vi "Add Panel.vi"(0 "Top Rack Serial Number":string, 1 "Work Order":string, 2 "Waveform":string, 3 "Frequency (MHz)":string, 4 "Bottom Rack Serial Number":string, 5 "Shelf Number":string, 6 "User":string, 7 "PartNumber":string, 8 "SubNumber":string, 9 "Voltage":string, 10 "connection information":path, 11 "System Num":u32=1 min=1 max=6) -> ()   [LabVIEW 2024]
uses:
  <vilib>/addons/database/Connection.llb/DB Tools Open Connec (Path).vi
  <vilib>/addons/database/Connection.llb/Conn Execute.vi
  <vilib>/addons/database/Recordset.llb/Rec Destroy - Connection.vi
  <vilib>/addons/database/_DB Variant To Data/Database Variant To Data.xnode
  <vilib>/addons/database/NI_Database_API.lvlib
panel:
  out "TimeStart":string
  out "Last DC_SN":string
  out "System #":u32=1 min=1 max=6
  in  "Active Positions 1":string
  in  "Active Positions 2":string
  out "Rack 2":string
  out "Rack 1":string
  in  "Deselect All 2":bool
  in  "Select All 2":bool
  in  "13":bool
  in  "14":bool
  in  "15":bool
  in  "16":bool
  in  "21":bool
  in  "22":bool
  in  "23":bool
  in  "24":bool
  in  "29":bool
  in  "30":bool
  in  "31":bool
  in  "32":bool
  in  "10":bool
  in  "11":bool
  in  "12":bool
  in  "18":bool
  in  "19":bool
  in  "20":bool
  in  "26":bool
  in  "27":bool
  in  "28":bool
  in  "1":bool
  in  "2":bool
  in  "3":bool
  in  "4":bool
  in  "5":bool
  in  "6":bool
  in  "7":bool
  in  "8":bool
  in  "9":bool
  in  "17":bool
  in  "25":bool
  in  "Deselect All 1":bool
  in  "Confirm":bool
  in  "13":bool
  in  "14":bool
  in  "15":bool
  in  "16":bool
  in  "21":bool
  in  "22":bool
  in  "23":bool
  in  "24":bool
  in  "29":bool
  in  "30":bool
  in  "31":bool
  in  "32":bool
  in  "10":bool
  in  "11":bool
  in  "12":bool
  in  "18":bool
  in  "19":bool
  in  "20":bool
  in  "26":bool
  in  "27":bool
  in  "28":bool
  in  "1":bool
  in  "2":bool
  in  "3":bool
  in  "4":bool
  in  "5":bool
  in  "6":bool
  in  "7":bool
  in  "8":bool
  in  "9":bool
  in  "17":bool
  in  "25":bool
  in  "Select All 1":bool
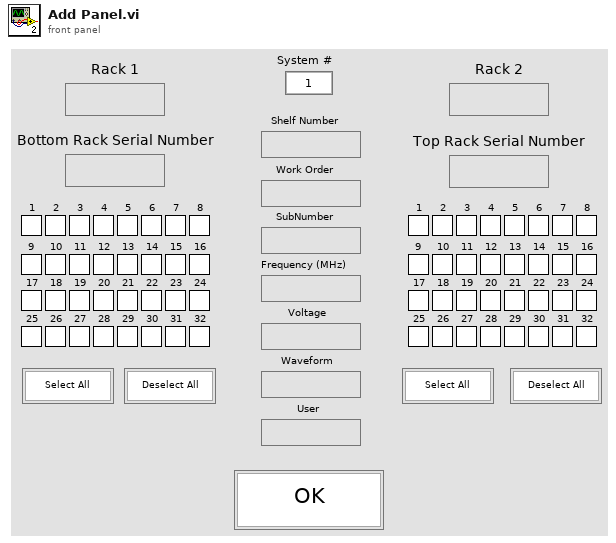
[diagram p1: front panel]
types:
  T1 = typedef "NI_Database_API.lvlib/Conn ObjectReference.ctl" = refnum<k1>
  T2 = typedef "NI_Database_API.lvlib/Rec ObjectReference.ctl" = refnum<k1>
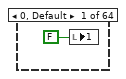
[diagram p2: hidden frame]
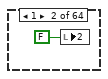
[diagram p3: hidden frame]
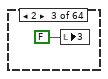
[diagram p4: hidden frame]
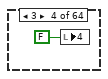
[diagram p5: hidden frame]
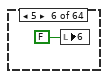
[diagram p6: hidden frame]
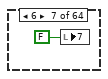
[diagram p7: hidden frame]
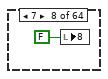
[diagram p8: hidden frame]
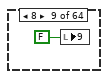
[diagram p9: hidden frame]
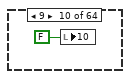
[diagram p10: hidden frame]
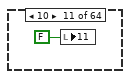
[diagram p11: hidden frame]
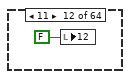
[diagram p12: hidden frame]
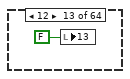
[diagram p13: hidden frame]
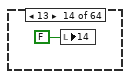
[diagram p14: hidden frame]
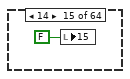
[diagram p15: hidden frame]
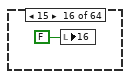
[diagram p16: hidden frame]
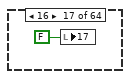
[diagram p17: hidden frame]
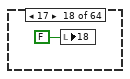
[diagram p18: hidden frame]
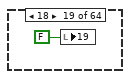
[diagram p19: hidden frame]
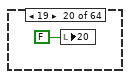
[diagram p20: hidden frame]
diagram:
  # "Any Questions? \nAsk Ben Wolford"
  n1 = flat-sequence {
    frame #0 {
      # "Opens SQL Active Systems/Racks/Positions and selects the data to show the user which positions are currently in use"
      n2 = property class="VI"() -> ("Front Panel"=w10:refnum<vi>)  [unwired: 2 in, 2 out]
      n3 = call "Display Message to User"() -> ()  [unwired: 10 in, 2 out]
      n4 = local write "Select All 1"(FALSE ("Select All")) -> ()
      n5 = local write "Confirm"(FALSE ("Confirm")) -> ()
      n6 = for {
        N: 64 -> [_]
        i -> [w13]
        n7 = case shown="4" w13 {
          frame 0, Default {
            n8 = local write "1"(FALSE ("1")) -> ()
          }
          frame 1 {
            n9 = local write "2"(FALSE ("1")) -> ()
          }
          frame 2 {
            n10 = local write "3"(FALSE ("1")) -> ()
          }
          frame 3 {
            n11 = local write "4"(FALSE ("1")) -> ()
          }
          frame 4 {
            n12 = local write "5"(FALSE ("1")) -> ()
          }
          frame 5 {
            n13 = local write "6"(FALSE ("1")) -> ()
          }
          frame 6 {
            n14 = local write "7"(FALSE ("1")) -> ()
          }
          frame 7 {
            n15 = local write "8"(FALSE ("1")) -> ()
          }
          frame 8 {
            n16 = local write "9"(FALSE ("1")) -> ()
          }
          frame 9 {
            n17 = local write "10"(FALSE ("1")) -> ()
          }
          frame 10 {
            n18 = local write "11"(FALSE ("1")) -> ()
          }
          frame 11 {
            n19 = local write "12"(FALSE ("1")) -> ()
          }
          frame 12 {
            n20 = local write "13"(FALSE ("1")) -> ()
          }
          frame 13 {
            n21 = local write "14"(FALSE ("1")) -> ()
          }
          frame 14 {
            n22 = local write "15"(FALSE ("1")) -> ()
          }
          frame 15 {
            n23 = local write "16"(FALSE ("1")) -> ()
          }
          frame 16 {
            n24 = local write "17"(FALSE ("1")) -> ()
          }
          frame 17 {
            n25 = local write "18"(FALSE ("1")) -> ()
          }
          frame 18 {
            n26 = local write "19"(FALSE ("1")) -> ()
          }
          frame 19 {
            n27 = local write "20"(FALSE ("1")) -> ()
          }
          frame 20 {
            n28 = local write "21"(FALSE ("1")) -> ()
          }
          frame 21 {
            n29 = local write "22"(FALSE ("1")) -> ()
          }
          frame 22 {
            n30 = local write "23"(FALSE ("1")) -> ()
          }
          frame 23 {
            n31 = local write "24"(FALSE ("1")) -> ()
          }
          frame 24 {
            n32 = local write "25"(FALSE ("1")) -> ()
          }
          frame 25 {
            n33 = local write "26"(FALSE ("1")) -> ()
          }
          frame 26 {
            n34 = local write "27"(FALSE ("1")) -> ()
          }
          frame 27 {
            n35 = local write "28"(FALSE ("1")) -> ()
          }
          frame 28 {
            n36 = local write "29"(FALSE ("1")) -> ()
          }
          frame 29 {
            n37 = local write "30"(FALSE ("1")) -> ()
          }
          frame 30 {
            n38 = local write "31"(FALSE ("1")) -> ()
          }
          frame 31 {
            n39 = local write "32"(FALSE ("1")) -> ()
          }
          frame 32 {
            n40 = local write "1"(FALSE ("1")) -> ()
          }
          frame 33 {
            n41 = local write "2"(FALSE ("1")) -> ()
          }
          frame 34 {
            n42 = local write "3"(FALSE ("1")) -> ()
          }
          frame 35 {
            n43 = local write "4"(FALSE ("1")) -> ()
          }
          frame 36 {
            n44 = local write "5"(FALSE ("1")) -> ()
          }
          frame 37 {
            n45 = local write "6"(FALSE ("1")) -> ()
          }
          frame 38 {
            n46 = local write "7"(FALSE ("1")) -> ()
          }
          frame 39 {
            n47 = local write "8"(FALSE ("1")) -> ()
          }
          frame 40 {
            n48 = local write "9"(FALSE ("1")) -> ()
          }
          frame 41 {
            n49 = local write "10"(FALSE ("1")) -> ()
          }
          frame 42 {
            n50 = local write "11"(FALSE ("1")) -> ()
          }
          frame 43 {
            n51 = local write "12"(FALSE ("1")) -> ()
          }
          frame 44 {
            n52 = local write "13"(FALSE ("1")) -> ()
          }
          frame 45 {
            n53 = local write "14"(FALSE ("1")) -> ()
          }
          frame 46 {
            n54 = local write "15"(FALSE ("1")) -> ()
          }
          frame 47 {
            n55 = local write "16"(FALSE ("1")) -> ()
          }
          frame 48 {
            n56 = local write "17"(FALSE ("1")) -> ()
          }
          frame 49 {
            n57 = local write "18"(FALSE ("1")) -> ()
          }
          frame 50 {
            n58 = local write "19"(FALSE ("1")) -> ()
          }
          frame 51 {
            n59 = local write "20"(FALSE ("1")) -> ()
          }
          frame 52 {
            n60 = local write "21"(FALSE ("1")) -> ()
          }
          frame 53 {
            n61 = local write "22"(FALSE ("1")) -> ()
          }
          frame 54 {
            n62 = local write "23"(FALSE ("1")) -> ()
          }
          frame 55 {
            n63 = local write "24"(FALSE ("1")) -> ()
          }
          frame 56 {
            n64 = local write "25"(FALSE ("1")) -> ()
          }
          frame 57 {
            n65 = local write "26"(FALSE ("1")) -> ()
          }
          frame 58 {
            n66 = local write "27"(FALSE ("1")) -> ()
          }
          frame 59 {
            n67 = local write "28"(FALSE ("1")) -> ()
          }
          frame 60 {
            n68 = local write "29"(FALSE ("1")) -> ()
          }
          frame 61 {
            n69 = local write "30"(FALSE ("1")) -> ()
          }
          frame 62 {
            n70 = local write "31"(FALSE ("1")) -> ()
          }
          frame 63 {
            n71 = local write "32"(FALSE ("1")) -> ()
          }
        }
      }
      n72 = property class="Pnl"(reference=w10, "Color"=u32 14869218) -> ()  [unwired: 1 in, 2 out]
      n73 = case shown="\"2\"" "Shelf Number" {
        tunnel: ["1" ("ConnectionString In") "3" ("ConnectionString In") "5" ("ConnectionString In") "7" ("ConnectionString In") "9" ("ConnectionString In") "11" ("ConnectionString In") "13" ("ConnectionString In") "15" ("ConnectionString In")] -> w7
        tunnel: ["2" ("ConnectionString In") "4" ("ConnectionString In") "6" ("ConnectionString In") "8" ("ConnectionString In") "10" ("ConnectionString In") "12" ("ConnectionString In") "14" ("ConnectionString In") "16" ("ConnectionString In")] -> w6
        frame "1", Default {
        }
        frame "2" {
        }
        frame "3" {
        }
        frame "4" {
        }
        frame "5" {
        }
        frame "6" {
        }
        frame "7" {
        }
        frame "8" {
        }
      }
      "Rack 1" <- w7
      "Rack 2" <- w6
      n74 = Get Date/Time In Seconds() -> (seconds since 1Jan1904=w3:timestamp)
      n75 = Format Date/Time String(time format string (%c)="%m/%d/%Y %I:%M %p", seconds (now)=w3) -> (date/time string=→"TimeStart":string)  [unwired: 1 in]
      "System #" <- "System Num"
    }
    frame #1 {
      n76 = while {
        stop <- w94 stop-if-true
        # "When deselect all is pressed down, set every button to inactive position"
        # "When Confirm is pressed, the current active positions are sent up to the cloud to save which ones are being used"
        # "When select all is pressed down, set every button to active position"
        n77 = event shown="[0] \"Confirm\": Value Change" {
          selector: _ -> [_ _ _ _ _]
          dyn-events: _ -> [_ _ _ _ _]
          timeout: _ -> [_ _ _ _ _]
          tunnel: [w103 _ _ _ _] -> w94
          event "Confirm": Value Change {
            n78 = event-data() -> ()  [unwired: 1 in, 1 out]
            n79 = flat-sequence {
              tunnel: [w138] -> w104
              tunnel: [w105] -> w102
              tunnel: w104 -> [w172]
              tunnel: w102 -> [w173]
              tunnel: [w175] -> w101
              tunnel: [w174] -> w100
              tunnel: w101 -> [w486]
              tunnel: w100 -> [w485]
              tunnel: [w480] -> w98
              tunnel: [w484] -> w96
              tunnel: [w599] -> w99
              tunnel: w98 -> [w599]
              tunnel: [w598] -> w97
              tunnel: w96 -> [w598]
              tunnel: w99 -> [w610]
              tunnel: w97 -> [w609]
              tunnel: [TRUE] -> w103
              frame #0 {
                # "Creates a Panel that allows users to click on individual positions to add them to the active positions"
                n80 = Build Array("1", "2", "3", "4", "5", "6", "7", "8", "9", "10", "11", "12", "13", "14", "15", "16", "17", "18", "19", "20", "21", "22", "23", "24", "25", "26", "27", "28", "29", "30", "31", "32") -> (w138:bool[])
                n81 = Build Array("1", "2", "3", "4", "5", "6", "7", "8", "9", "10", "11", "12", "13", "14", "15", "16", "17", "18", "19", "20", "21", "22", "23", "24", "25", "26", "27", "28", "29", "30", "31", "32") -> (w105:bool[])
              }
              frame #1 {
                n82 = Or Array Elements(Boolean array=w172) -> (logical OR=w177:bool)
                n83 = Or Array Elements(Boolean array=w173) -> (logical OR=w176:bool)
                n84 = Insert Into Array(array=w172, new element=w173) -> (w171:bool[])  [unwired: 1 in]
                n85 = Not(x=w177) -> (.not. x?=w175:bool)
                n86 = for {
                  N: 64 -> [_]
                  tunnel: w171 -> [w180] mode=indexing
                  shift-right: [w182] -> _
                  shift-left: "" -> [w191]
                  i -> [w187]
                  n87 = Select(t="1", s=w180, f="0") -> (s? t:f=w186:string)
                  n88 = Increment(x=w187) -> (x+1=w183:i32)
                  n89 = Concatenate Strings(w191, w186, "," ("string")) -> (w185:string)
                  n90 = Greater?(x=w183, y=32) -> (0:w181:bool)
                  n91 = case shown="True" w180 {
                    tunnel: w183 -> [_ w224]
                    tunnel: w181 -> [_ w223]
                    frame False {
                    }
                    frame True {
                      n92 = flat-sequence {
                        tunnel: w224 -> [w254]
                        tunnel: [w245] -> w216
                        tunnel: [w246] -> w214
                        tunnel: [w257] -> w212
                        tunnel: [w288] -> w210
                        tunnel: [w287] -> w208
                        tunnel: [w261] -> w206
                        tunnel: w223 -> [w253]
                        tunnel: [w245] -> w204
                        tunnel: w216 -> [w385]
                        tunnel: [w385] -> w215
                        tunnel: w214 -> [w384]
                        tunnel: [w384] -> w213
                        tunnel: w212 -> [w383]
                        tunnel: [w383] -> w211
                        tunnel: w210 -> [w382]
                        tunnel: [w382] -> w209
                        tunnel: w208 -> [w381]
                        tunnel: [w381] -> w207
                        tunnel: w206 -> [w380]
                        tunnel: [w380] -> w205
                        tunnel: w204 -> [w379]
                        tunnel: [w379] -> w203
                        tunnel: w215 -> [w395]
                        tunnel: [w395] -> w222
                        tunnel: w213 -> [w394]
                        tunnel: [w394] -> w221
                        tunnel: w211 -> [w393]
                        tunnel: [w393] -> w220
                        tunnel: w209 -> [w392]
                        tunnel: [w392] -> w219
                        tunnel: w207 -> [w391]
                        tunnel: [w391] -> w218
                        tunnel: w205 -> [w389]
                        tunnel: [w389] -> w217
                        tunnel: w203 -> [w386]
                        tunnel: w222 -> [_]
                        tunnel: w221 -> [_]
                        tunnel: w220 -> [_]
                        tunnel: w219 -> [w404]
                        tunnel: w218 -> [w405]
                        tunnel: w217 -> [w426]
                        frame #0 {
                          w243 = "," ("string")
                          # "If true, the DC_SN is checked that it abides by the format, and adds all the data displayed in the master key for the oscillator"
                          # "Master Key:\n1. DC_SN\n2. WorkOrder\n3. SystemNumber\n4. RackNumber\n5. PositionNumber\n6. RackSerialNumber\n7. TimeStart\n8. Nominal Frequency\n9. OscVoltage\n10. Waveform"
                          n93 = while {
                            tunnel: [w316] -> w246
                            stop <- w315 stop-if-true
                            n94 = flat-sequence {
                              tunnel: [w318] -> w314
                              tunnel: [w317] -> w313
                              tunnel: [w326] -> w312
                              tunnel: [w323] -> w310
                              tunnel: [w324] -> w308
                              tunnel: w313 -> [w325]
                              tunnel: w314 -> [w326]
                              tunnel: w312 -> [w370]
                              tunnel: [w370] -> w311
                              tunnel: w310 -> [w369]
                              tunnel: [w369] -> w309
                              tunnel: w308 -> [w368]
                              tunnel: w311 -> [w375]
                              tunnel: [w375] -> w316
                              tunnel: w309 -> [w372]
                              tunnel: [w373] -> w315
                              frame #0 {
                                n95 = call "Prompt User for Input"() -> ("DC_SN"=w318:string)  [unwired: 17 in, 2 out]
                                n96 = String To Byte Array(string=w318) -> (unsigned byte array=w317:u8[])
                              }
                              frame #1 {
                                n97 = Index Array(array=w325, index=0) -> (element=w319:u8)
                                n98 = Not Equal?(x=69, y=w319) -> (x != y?=w321:bool)
                                n99 = case shown="False" w321 {
                                tunnel: w326 -> [_ w347]
                                tunnel: [w327 w345] -> w324
                                tunnel: w325 -> [w330 w343]
                                tunnel: w319 -> [_ w338]
                                frame False {
                                n100 = Array Subset(array=w330, index=1) -> (w329:u8[])  [unwired: 1 in]
                                n101 = for {
                                N: 5 -> [_]
                                tunnel: w329 -> [w337] mode=indexing
                                tunnel: [w333] -> w328 mode=indexing
                                n102 = In Range and Coerce(upper limit=u8 57, x=w337, lower limit=u8 48) -> (In Range?=w334:bool)  [unwired: 1 out]
                                n103 = Not(x=w334) -> (.not. x?=w333:bool)
                                }
                                n104 = Or Array Elements(Boolean array=w328) -> (logical OR=w327:bool)
                                }
                                frame True {
                                n105 = String Length(string=w347) -> (length=w353:i32)
                                n106 = Equal?(x=u8 66, y=w338) -> (x = y?=w341:bool)
                                n107 = Equal?(x=u8 98, y=w338) -> (x = y?=w339:bool)
                                n108 = Or(x=w341, y=w339) -> (x .or. y?=w342:bool)
                                n109 = case shown="False" w342 {
                                tunnel: w343 -> [w364 w367]
                                tunnel: [w364 w365] -> w346
                                frame False {
                                }
                                frame True {
                                n110 = Array Subset(array=w367, index=1) -> (w365:u8[])  [unwired: 1 in]
                                }
                                }
                                n111 = Not Equal?(x=10, y=w353) -> (x != y?=w354:bool)
                                n112 = Array Max & Min(array=w346) -> (max value=w359:u8, min value=w358:u8)  [unwired: 2 out]
                                n113 = Index Array(array=w346, index=4) -> (element=w355:u8)
                                n114 = Less Or Equal?(x=w359, y=u8 57) -> (x <= y?=w360:bool)
                                n115 = Greater Or Equal?(x=w358, y=u8 46) -> (x >= y?=w361:bool)
                                n116 = And(x=w360, y=w361) -> (x .and. y?=w362:bool)
                                n117 = Not Equal?(x=w355, y=u8 46) -> (x != y?=w357:bool)
                                n118 = Not(x=w362) -> (.not. x?=w363:bool)
                                n119 = Or(x=w357, y=w363) -> (x .or. y?=w356:bool)
                                n120 = Or(x=w354, y=w356) -> (x .or. y?=w345:bool)
                                }
                                }
                                n121 = Not(x=w324) -> (.not. x?=w323:bool)
                              }
                              frame #2 {
                                n122 = call "Display Message to User"("Enable"=w368) -> ()  [unwired: 9 in, 2 out]
                              }
                              frame #3 {
                                n123 = Concatenate Strings("You entered " ("string"), w375, " is this correct?" ("string")) -> (w371:string)
                                n124 = call "Display Message to User"("Enable"=w372, "Message"=w371) -> ("Yes"=w374:bool)  [unwired: 8 in, 1 out]
                                n125 = And(x=w374, y=w372) -> (x .and. y?=w373:bool)
                              }
                            }
                          }
                          n126 = Random Number (0-1)() -> (number: 0 to 1=w235:dbl)
                          n127 = case shown="False" w253 {
                            tunnel: [w302 w307] -> w247
                            tunnel: w254 -> [w301 w306]
                            tunnel: [w301 w304] -> w255
                            tunnel: [w300 w303] -> w252
                            frame False {
                              n128 = local read "Bottom Rack Serial Number"() -> (w300:string)
                              n129 = local read "Rack 1"() -> (w302:string)
                            }
                            frame True {
                              n130 = Subtract(x=w306, y=32) -> (x-y=w304:i32)
                              n131 = local read "Top Rack Serial Number"() -> (w303:string)
                              n132 = local read "Rack 2"() -> (w307:string)
                            }
                          }
                          n133 = Multiply(x=51.0, y=w235) -> (x*y=w232:dbl)
                          n134 = Greater?(x=w232, y=25.0) -> (0:w230:bool)
                          n135 = case shown="True" w230 {
                            tunnel: w232 -> [w296 w299]
                            tunnel: [w296 w297] -> w231
                            frame False {
                            }
                            frame True {
                              n136 = Add(x=w299, y=7.0) -> (x+y=w297:dbl)
                            }
                          }
                          n137 = Add(x=w231, y=65.0) -> (x+y=w229:dbl)
                          n138 = local read "System Num"() -> (w289:u32)
                          n139 = Build Array(w229) -> (w228:dbl[])
                          n140 = local read "Frequency (MHz)"() -> (w269:string)
                          n141 = local read "Work Order"() -> (w295:string)
                          n142 = local read "SubNumber"() -> (w258:string)
                          n143 = local read "PartNumber"() -> (w240:string)
                          n144 = local read "Waveform"() -> (w273:string)
                          n145 = local read "TimeStart"() -> (w225:string)
                          n146 = local read "Voltage"() -> (w271:string)
                          n147 = local read "User"() -> (w249:string)
                          n148 = To Unsigned Byte Integer(number=w228) -> (unsigned 8bit integer=w227:u8[])
                          n149 = Number To Decimal String(number=w289) -> (decimal integer string=w284:string)  [unwired: 1 in]
                          n150 = Number To Decimal String(number=w255) -> (decimal integer string=w263:string)  [unwired: 1 in]
                          n151 = Concatenate Strings("'" ("string"), w247, "'" ("string")) -> (w280:string)
                          n152 = Byte Array To String(unsigned byte array=w227) -> (string=w226:string)
                          n153 = Concatenate Strings("'" ("string"), w295, "'" ("string")) -> (w257:string)
                          n154 = Concatenate Strings("'" ("string"), w258, "'" ("string")) -> (w256:string)
                          n155 = Concatenate Strings("'" ("string"), w284, "'" ("string")) -> (w283:string)
                          n156 = Concatenate Strings("'" ("string"), w263, "'" ("string")) -> (w245:string)
                          n157 = Concatenate Strings("'" ("string"), w225, "'" ("string")) -> (w294:string)
                          n158 = Concatenate Strings("'" ("string"), w269, "'" ("string")) -> (w268:string)
                          n159 = Concatenate Strings("'" ("string"), w271, "'" ("string")) -> (w270:string)
                          n160 = Concatenate Strings("'" ("string"), w273, "'" ("string")) -> (w272:string)
                          n161 = Concatenate Strings("'" ("string"), w249, "'" ("string")) -> (w248:string)
                          n162 = Concatenate Strings("'" ("string"), w240, "'" ("string")) -> (w239:string)
                          n163 = Concatenate Strings("'" ("string"), w246, "'" ("string")) -> (w261:string)
                          n164 = Concatenate Strings("UPDATE MASTER\nSET DC_SN = CONCAT(DC_SN, '" ("string"), w226, "')\nWHERE DC_SN = " ("string"), w261) -> (w287:string)
                          n165 = Concatenate Strings("INSERT INTO MASTER\nVALUES(" ("SQL Query"), w261, w243, w257, w243, w256, w243, w283, w243, w280, w243, w245, w243, w252, w243, w294, w243, w268, w243, w270, w243, w272, w243, w248, w243, w239, ");" ("string")) -> (w288:string)
                        }
                        frame #1 {
                          n166 = Wait (ms)(milliseconds to wait=u32 500) -> ()  [unwired: 1 out]
                        }
                        frame #2 {
                          n167 = Concatenate Strings("Please place DC_SN " ("Message"), w389, " into position " ("string"), w386) -> (w387:string)
                          n168 = call "Display Message to User"("Message"=w387) -> ()  [unwired: 9 in, 2 out]
                        }
                        frame #3 {
                          n169 = local read "connection information"() -> (w413:path)
                          n170 = Concatenate Strings("WHERE DC_SN = " ("SQL Query"), w426) -> (w407:string)
                          n171 = call-poly <vilib>:"DB Tools Open Connection.vi"("connection information"=w413) -> ("error out"=w414:errorcluster, "connection reference"=w417:T1)  [unwired: 7 in]
                          n172 = call <vilib>:"DB Tools Select Data.vi"("condition"=w407, "error in (no error)"=w414, "table"="MASTER", "connection reference"=w417) -> ("error out"=w412:errorcluster, "data"=w410:variant[][], "connection reference out"=w416:T1)  [unwired: 2 in]
                          n173 = xnode "Database Variant To Data"("database variant"=w410, "error in (no error)"=w412, "type"=string[][] [] ("ConnectionString In")) -> ("data"=w406:string[][], "error out"=w411:errorcluster)
                          n174 = Array Size(array=w406) -> (size(s)=w425:i32[])
                          n175 = Index Array(array=w425, index=0) -> (element=w422:i32)
                          n176 = Index Array(array=w425, index=1) -> (element=w397:i32)
                          n177 = Greater?(x=w422, y=0) -> (0:w420:bool)
                          n178 = Greater?(x=w397, y=0) -> (0:w419:bool)
                          n179 = And(x=w420, y=w419) -> (x .and. y?=w403:bool)
                          n180 = case shown="True" w403 {
                            tunnel: w416 -> [w427 w435]
                            tunnel: [w428 w430] -> w415
                            tunnel: w411 -> [w428 w434]
                            tunnel: w405 -> [_ w433]
                            tunnel: [w427 w431] -> w402
                            frame False {
                            }
                            frame True {
                              n181 = call-poly <vilib>:"DB Tools Execute Query.vi"("error in (no error)"=w434, "SQL query"=w433, "connection reference"=w435) -> ("error out"=w429:errorcluster, "recordset reference"=w432:T2)  [unwired: 5 in]
                              n182 = call-poly <vilib>:"DB Tools Free Object.vi"("error in (no error)"=w429, "recordset reference"=w432) -> ("error out"=w430:errorcluster, "connection reference"=w431:T1)  [unwired: 8 in]
                            }
                          }
                          n183 = call-poly <vilib>:"DB Tools Execute Query.vi"("error in (no error)"=w415, "SQL query"=w404, "connection reference"=w402) -> ("error out"=w400:errorcluster, "recordset reference"=w401:T2)  [unwired: 5 in]
                          n184 = call-poly <vilib>:"DB Tools Free Object.vi"("error in (no error)"=w400, "recordset reference"=w401) -> ("error out"=w398:errorcluster, "connection reference"=w399:T1)  [unwired: 8 in]
                          n185 = call <vilib>:"DB Tools Close Connection.vi"("error in (no error)"=w398, "connection reference"=w399) -> ()  [unwired: 5 in, 1 out]
                        }
                      }
                    }
                  }
                  n186 = case shown="0, Default" w183 {
                    tunnel: w185 -> [w192 w199 w202]
                    tunnel: ["" "" w202] -> w182
                    tunnel: w181 -> [_ _ _]
                    frame 64 {
                      n187 = String Length(string=w192) -> (length=w195:i32)
                      n188 = Decrement(x=w195) -> (x-1=w196:i32)
                      n189 = String Subset(string=w192, length (rest)=w196) -> (substring=w194:string)  [unwired: 1 in]
                      n190 = local write "Active Positions 2"(w194) -> ()
                    }
                    frame 32 {
                      n191 = String Length(string=w199) -> (length=w200:i32)
                      n192 = Decrement(x=w200) -> (x-1=w201:i32)
                      n193 = String Subset(string=w199, length (rest)=w201) -> (substring=w198:string)  [unwired: 1 in]
                      n194 = local write "Active Positions 1"(w198) -> ()
                    }
                    frame 0, Default {
                    }
                  }
                }
                n195 = Not(x=w176) -> (.not. x?=w174:bool)
              }
              frame #2 {
                n196 = Or(x=w486, y=w485) -> (x .or. y?=w487:bool)
                n197 = local read "connection information"() -> (w482:path)
                n198 = call-poly <vilib>:"DB Tools Open Connection.vi"("connection information"=w482) -> ("error out"=w483:errorcluster, "connection reference"=w481:T1)  [unwired: 7 in]
                n199 = case shown="True" w487 {
                  tunnel: w486 -> [_ w497]
                  tunnel: w483 -> [w489 w495]
                  tunnel: [w489 w490] -> w484
                  tunnel: w481 -> [w488 w496]
                  tunnel: [w488 w493] -> w480
                  frame False {
                  }
                  frame True {
                    n200 = case shown="False" w497 {
                      tunnel: [w510 w560] -> w494
                      frame False {
                        n201 = local read "System Num"() -> (w498:u32)
                        n202 = local read "Rack 2"() -> (w503:string)
                        n203 = Fract/Exp String To Number(string=w503) -> (number=w502:dbl)  [unwired: 3 in, 1 out]
                        n204 = Number To Decimal String(number=w498) -> (decimal integer string=w499:string)  [unwired: 1 in]
                        n205 = case shown="4" w502 {
                          tunnel: [w516 w520 w524 w528 w532 w537 w540 w544] -> w501
                          tunnel: w499 -> [w517 w521 w525 w529 w533 w536 w541 w545]
                          frame 2, Default {
                            n206 = Concatenate Strings("A", w517, ".2") -> (w516:string)
                          }
                          frame 4 {
                            n207 = Concatenate Strings("A", w521, ".4") -> (w520:string)
                          }
                          frame 6 {
                            n208 = Concatenate Strings("A", w525, ".6") -> (w524:string)
                          }
                          frame 8 {
                            n209 = Concatenate Strings("A", w529, ".8") -> (w528:string)
                          }
                          frame 10 {
                            n210 = Concatenate Strings("A", w533, ".10") -> (w532:string)
                          }
                          frame 12 {
                            n211 = Concatenate Strings("A", w536, ".12") -> (w537:string)
                          }
                          frame 14 {
                            n212 = Concatenate Strings("A", w541, ".14") -> (w540:string)
                          }
                          frame 16 {
                            n213 = Concatenate Strings("A", w545, ".16") -> (w544:string)
                          }
                        }
                        n214 = local read "Top Rack Serial Number"() -> (w504:string)
                        n215 = Get Date/Time In Seconds() -> (seconds since 1Jan1904=w511:timestamp)
                        n216 = Format Date/Time String(time format string (%c)="%m/%d/%Y %I:%M %p", seconds (now)=w511) -> (date/time string=w512:string)  [unwired: 1 in]
                        n217 = Concatenate Strings("'" ("string"), w512, "'" ("string")) -> (w506:string)
                        n218 = Concatenate Strings("UPDATE MASTER\nSet TimeStart = " ("string"), w506, ", RackSerialNumber = " ("string"), w504, "WHERE RackNumber = " ("string"), w503, " AND DC_SN = '" ("string"), w501, "'" ("string")) -> (w510:string)
                      }
                      frame True {
                        n219 = local read "System Num"() -> (w549:u32)
                        n220 = local read "Rack 1"() -> (w553:string)
                        n221 = Fract/Exp String To Number(string=w553) -> (number=w552:dbl)  [unwired: 3 in, 1 out]
                        n222 = Number To Decimal String(number=w549) -> (decimal integer string=w548:string)  [unwired: 1 in]
                        n223 = case shown="1, Default" w552 {
                          tunnel: [w566 w570 w574 w578 w582 w586 w590 w595] -> w551
                          tunnel: w548 -> [w567 w571 w575 w579 w583 w587 w591 w594]
                          frame 1, Default {
                            n224 = Concatenate Strings("A", w567, ".1") -> (w566:string)
                          }
                          frame 3 {
                            n225 = Concatenate Strings("A", w571, ".3") -> (w570:string)
                          }
                          frame 5 {
                            n226 = Concatenate Strings("A", w575, ".5") -> (w574:string)
                          }
                          frame 7 {
                            n227 = Concatenate Strings("A", w579, ".7") -> (w578:string)
                          }
                          frame 9 {
                            n228 = Concatenate Strings("A", w583, ".9") -> (w582:string)
                          }
                          frame 11 {
                            n229 = Concatenate Strings("A", w587, ".11") -> (w586:string)
                          }
                          frame 13 {
                            n230 = Concatenate Strings("A", w591, ".13") -> (w590:string)
                          }
                          frame 15 {
                            n231 = Concatenate Strings("A", w594, ".15") -> (w595:string)
                          }
                        }
                        n232 = local read "Bottom Rack Serial Number"() -> (w554:string)
                        n233 = Get Date/Time In Seconds() -> (seconds since 1Jan1904=w561:timestamp)
                        n234 = Format Date/Time String(time format string (%c)="%m/%d/%Y %I:%M %p", seconds (now)=w561) -> (date/time string=w562:string)  [unwired: 1 in]
                        n235 = Concatenate Strings("'" ("string"), w562, "'" ("string")) -> (w556:string)
                        n236 = Concatenate Strings("UPDATE MASTER\nSet TimeStart = " ("string"), w556, ", RackSerialNumber = " ("string"), w554, "WHERE RackNumber = " ("string"), w553, " AND DC_SN = '" ("string"), w551, "'" ("string")) -> (w560:string)
                      }
                    }
                    n237 = call-poly <vilib>:"DB Tools Execute Query.vi"("error in (no error)"=w495, "SQL query"=w494, "connection reference"=w496) -> ("error out"=w491:errorcluster, "recordset reference"=w492:T2)  [unwired: 5 in]
                    n238 = call-poly <vilib>:"DB Tools Free Object.vi"("error in (no error)"=w491, "recordset reference"=w492) -> ("error out"=w490:errorcluster, "connection reference"=w493:T1)  [unwired: 8 in]
                  }
                }
              }
              frame #3 {
                n239 = Wait (ms)(milliseconds to wait=u32 500) -> ()  [unwired: 1 out]
              }
              frame #4 {
                w615 = "   AND Rack = " ("SQL Query")
                w617 = "WHERE System = " ("SQL Query")
                w613 = ";" ("string")
                w618 = "UPDATE ACTIVE\nSET Position = " ("SQL Query")
                # "Removes the old string in active with the current string that has the positions added"
                n240 = local read "System Num"() -> (w631:u32)
                n241 = Number To Decimal String(number=w631) -> (decimal integer string=w624:string)  [unwired: 1 in]
                n242 = Concatenate Strings("'" ("string"), "Active Positions 2", "'\n" ("string")) -> (w619:string)
                n243 = Concatenate Strings("'" ("string"), "Active Positions 1", "'\n" ("string")) -> (w627:string)
                n244 = Concatenate Strings("'" ("string"), w624, "'" ("string")) -> (w616:string)
                n245 = local read "Rack 2"() -> (w614:string)
                n246 = local read "Rack 1"() -> (w623:string)
                n247 = Concatenate Strings(w618, w619, w617, w616, w615, w614, w613) -> (w611:string)
                n248 = Concatenate Strings(w618, w627, w617, w616, w615, w623, w613) -> (w612:string)
                n249 = call-poly <vilib>:"DB Tools Execute Query.vi"("error in (no error)"=w609, "SQL query"=w612, "connection reference"=w610) -> ("error out"=w608:errorcluster, "recordset reference"=w607:T2)  [unwired: 5 in]
                n250 = call-poly <vilib>:"DB Tools Free Object.vi"("error in (no error)"=w608, "recordset reference"=w607) -> ("error out"=w605:errorcluster, "connection reference"=w606:T1)  [unwired: 8 in]
                n251 = call-poly <vilib>:"DB Tools Execute Query.vi"("error in (no error)"=w605, "SQL query"=w611, "connection reference"=w606) -> ("error out"=w603:errorcluster, "recordset reference"=w604:T2)  [unwired: 5 in]
                n252 = call-poly <vilib>:"DB Tools Free Object.vi"("error in (no error)"=w603, "recordset reference"=w604) -> ("error out"=w601:errorcluster, "connection reference"=w602:T1)  [unwired: 8 in]
                n253 = call <vilib>:"DB Tools Close Connection.vi"("error in (no error)"=w601, "connection reference"=w602) -> ()  [unwired: 5 in, 1 out]
              }
              frame #5 {
              }
            }
          }
          event "Select All 1": Value Change {
            # "Turns all of the buttons/positions to true"
            n254 = event-data() -> ()  [unwired: 1 in, 3 out]
            n255 = stacked-sequence {
              frame #0 {
                n256 = local write "1"(TRUE) -> ()
              }
              frame #1 {
                n257 = local write "2"(TRUE) -> ()
              }
              frame #2 {
                n258 = local write "3"(TRUE) -> ()
              }
              frame #3 {
                n259 = local write "4"(TRUE) -> ()
              }
              frame #4 {
                n260 = local write "5"(TRUE) -> ()
              }
              frame #5 {
                n261 = local write "6"(TRUE) -> ()
              }
              frame #6 {
                n262 = local write "7"(TRUE) -> ()
              }
              frame #7 {
                n263 = local write "8"(TRUE) -> ()
              }
              frame #8 {
                n264 = local write "9"(TRUE) -> ()
              }
              frame #9 {
                n265 = local write "10"(TRUE) -> ()
              }
              frame #10 {
                n266 = local write "11"(TRUE) -> ()
              }
              frame #11 {
                n267 = local write "12"(TRUE) -> ()
              }
              frame #12 {
                n268 = local write "13"(TRUE) -> ()
              }
              frame #13 {
                n269 = local write "14"(TRUE) -> ()
              }
              frame #14 {
                n270 = local write "15"(TRUE) -> ()
              }
              frame #15 {
                n271 = local write "16"(TRUE) -> ()
              }
              frame #16 {
                n272 = local write "17"(TRUE) -> ()
              }
              frame #17 {
                n273 = local write "18"(TRUE) -> ()
              }
              frame #18 {
                n274 = local write "19"(TRUE) -> ()
              }
              frame #19 {
                n275 = local write "20"(TRUE) -> ()
              }
              frame #20 {
                n276 = local write "21"(TRUE) -> ()
              }
              frame #21 {
                n277 = local write "22"(TRUE) -> ()
              }
              frame #22 {
                n278 = local write "23"(TRUE) -> ()
              }
              frame #23 {
                n279 = local write "24"(TRUE) -> ()
              }
              frame #24 {
                n280 = local write "25"(TRUE) -> ()
              }
              frame #25 {
                n281 = local write "26"(TRUE) -> ()
              }
              frame #26 {
                n282 = local write "27"(TRUE) -> ()
              }
              frame #27 {
                n283 = local write "28"(TRUE) -> ()
              }
              frame #28 {
                n284 = local write "29"(TRUE) -> ()
              }
              frame #29 {
                n285 = local write "30"(TRUE) -> ()
              }
              frame #30 {
                n286 = local write "31"(TRUE) -> ()
              }
              frame #31 {
                n287 = local write "32"(TRUE) -> ()
              }
            }
          }
          event "Select All 2": Value Change {
            # "Turns all of the buttons/positions to true"
            n288 = event-data() -> ()  [unwired: 1 in, 3 out]
            n289 = stacked-sequence {
              frame #0 {
                n290 = local write "1"(TRUE) -> ()
              }
              frame #1 {
                n291 = local write "2"(TRUE) -> ()
              }
              frame #2 {
                n292 = local write "3"(TRUE) -> ()
              }
              frame #3 {
                n293 = local write "4"(TRUE) -> ()
              }
              frame #4 {
                n294 = local write "5"(TRUE) -> ()
              }
              frame #5 {
                n295 = local write "6"(TRUE) -> ()
              }
              frame #6 {
                n296 = local write "7"(TRUE) -> ()
              }
              frame #7 {
                n297 = local write "8"(TRUE) -> ()
              }
              frame #8 {
                n298 = local write "9"(TRUE) -> ()
              }
              frame #9 {
                n299 = local write "10"(TRUE) -> ()
              }
              frame #10 {
                n300 = local write "11"(TRUE) -> ()
              }
              frame #11 {
                n301 = local write "12"(TRUE) -> ()
              }
              frame #12 {
                n302 = local write "13"(TRUE) -> ()
              }
              frame #13 {
                n303 = local write "14"(TRUE) -> ()
              }
              frame #14 {
                n304 = local write "15"(TRUE) -> ()
              }
              frame #15 {
                n305 = local write "16"(TRUE) -> ()
              }
              frame #16 {
                n306 = local write "17"(TRUE) -> ()
              }
              frame #17 {
                n307 = local write "18"(TRUE) -> ()
              }
              frame #18 {
                n308 = local write "19"(TRUE) -> ()
              }
              frame #19 {
                n309 = local write "20"(TRUE) -> ()
              }
              frame #20 {
                n310 = local write "21"(TRUE) -> ()
              }
              frame #21 {
                n311 = local write "22"(TRUE) -> ()
              }
              frame #22 {
                n312 = local write "23"(TRUE) -> ()
              }
              frame #23 {
                n313 = local write "24"(TRUE) -> ()
              }
              frame #24 {
                n314 = local write "25"(TRUE) -> ()
              }
              frame #25 {
                n315 = local write "26"(TRUE) -> ()
              }
              frame #26 {
                n316 = local write "27"(TRUE) -> ()
              }
              frame #27 {
                n317 = local write "28"(TRUE) -> ()
              }
              frame #28 {
                n318 = local write "29"(TRUE) -> ()
              }
              frame #29 {
                n319 = local write "30"(TRUE) -> ()
              }
              frame #30 {
                n320 = local write "31"(TRUE) -> ()
              }
              frame #31 {
                n321 = local write "32"(TRUE) -> ()
              }
            }
          }
          event "Deselect All 1": Value Change {
            # "Turns all of the buttons/positions to false"
            n322 = event-data() -> ()  [unwired: 1 in, 3 out]
            n323 = stacked-sequence {
              frame #0 {
                n324 = local write "1"(FALSE) -> ()
              }
              frame #1 {
                n325 = local write "2"(FALSE) -> ()
              }
              frame #2 {
                n326 = local write "3"(FALSE) -> ()
              }
              frame #3 {
                n327 = local write "4"(FALSE) -> ()
              }
              frame #4 {
                n328 = local write "5"(FALSE) -> ()
              }
              frame #5 {
                n329 = local write "6"(FALSE) -> ()
              }
              frame #6 {
                n330 = local write "7"(FALSE) -> ()
              }
              frame #7 {
                n331 = local write "8"(FALSE) -> ()
              }
              frame #8 {
                n332 = local write "9"(FALSE) -> ()
              }
              frame #9 {
                n333 = local write "10"(FALSE) -> ()
              }
              frame #10 {
                n334 = local write "11"(FALSE) -> ()
              }
              frame #11 {
                n335 = local write "12"(FALSE) -> ()
              }
              frame #12 {
                n336 = local write "13"(FALSE) -> ()
              }
              frame #13 {
                n337 = local write "14"(FALSE) -> ()
              }
              frame #14 {
                n338 = local write "15"(FALSE) -> ()
              }
              frame #15 {
                n339 = local write "16"(FALSE) -> ()
              }
              frame #16 {
                n340 = local write "17"(FALSE) -> ()
              }
              frame #17 {
                n341 = local write "18"(FALSE) -> ()
              }
              frame #18 {
                n342 = local write "19"(FALSE) -> ()
              }
              frame #19 {
                n343 = local write "20"(FALSE) -> ()
              }
              frame #20 {
                n344 = local write "21"(FALSE) -> ()
              }
              frame #21 {
                n345 = local write "22"(FALSE) -> ()
              }
              frame #22 {
                n346 = local write "23"(FALSE) -> ()
              }
              frame #23 {
                n347 = local write "24"(FALSE) -> ()
              }
              frame #24 {
                n348 = local write "25"(FALSE) -> ()
              }
              frame #25 {
                n349 = local write "26"(FALSE) -> ()
              }
              frame #26 {
                n350 = local write "27"(FALSE) -> ()
              }
              frame #27 {
                n351 = local write "28"(FALSE) -> ()
              }
              frame #28 {
                n352 = local write "29"(FALSE) -> ()
              }
              frame #29 {
                n353 = local write "30"(FALSE) -> ()
              }
              frame #30 {
                n354 = local write "31"(FALSE) -> ()
              }
              frame #31 {
                n355 = local write "32"(FALSE) -> ()
              }
            }
          }
          event "Deselect All 2": Value Change {
            # "Turns all of the buttons/positions to false"
            n356 = event-data() -> ()  [unwired: 1 in, 3 out]
            n357 = stacked-sequence {
              frame #0 {
                n358 = local write "1"(FALSE) -> ()
              }
              frame #1 {
                n359 = local write "2"(FALSE) -> ()
              }
              frame #2 {
                n360 = local write "3"(FALSE) -> ()
              }
              frame #3 {
                n361 = local write "4"(FALSE) -> ()
              }
              frame #4 {
                n362 = local write "5"(FALSE) -> ()
              }
              frame #5 {
                n363 = local write "6"(FALSE) -> ()
              }
              frame #6 {
                n364 = local write "7"(FALSE) -> ()
              }
              frame #7 {
                n365 = local write "8"(FALSE) -> ()
              }
              frame #8 {
                n366 = local write "9"(FALSE) -> ()
              }
              frame #9 {
                n367 = local write "10"(FALSE) -> ()
              }
              frame #10 {
                n368 = local write "11"(FALSE) -> ()
              }
              frame #11 {
                n369 = local write "12"(FALSE) -> ()
              }
              frame #12 {
                n370 = local write "13"(FALSE) -> ()
              }
              frame #13 {
                n371 = local write "14"(FALSE) -> ()
              }
              frame #14 {
                n372 = local write "15"(FALSE) -> ()
              }
              frame #15 {
                n373 = local write "16"(FALSE) -> ()
              }
              frame #16 {
                n374 = local write "17"(FALSE) -> ()
              }
              frame #17 {
                n375 = local write "18"(FALSE) -> ()
              }
              frame #18 {
                n376 = local write "19"(FALSE) -> ()
              }
              frame #19 {
                n377 = local write "20"(FALSE) -> ()
              }
              frame #20 {
                n378 = local write "21"(FALSE) -> ()
              }
              frame #21 {
                n379 = local write "22"(FALSE) -> ()
              }
              frame #22 {
                n380 = local write "23"(FALSE) -> ()
              }
              frame #23 {
                n381 = local write "24"(FALSE) -> ()
              }
              frame #24 {
                n382 = local write "25"(FALSE) -> ()
              }
              frame #25 {
                n383 = local write "26"(FALSE) -> ()
              }
              frame #26 {
                n384 = local write "27"(FALSE) -> ()
              }
              frame #27 {
                n385 = local write "28"(FALSE) -> ()
              }
              frame #28 {
                n386 = local write "29"(FALSE) -> ()
              }
              frame #29 {
                n387 = local write "30"(FALSE) -> ()
              }
              frame #30 {
                n388 = local write "31"(FALSE) -> ()
              }
              frame #31 {
                n389 = local write "32"(FALSE) -> ()
              }
            }
          }
        }
        n390 = Wait (ms)(milliseconds to wait=u32 100) -> ()  [unwired: 1 out]
      }
    }
  }
